vi "Radio Button Value.vi"(8 "Error In":errorcluster, 10 "Radio Buttons 2":refnum<vi>) -> (0 "Error Out":errorcluster, 2 "1st Value Selected?":bool)   [LabVIEW 2016]
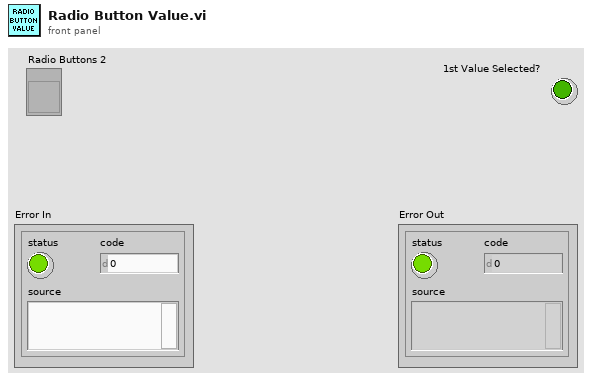
[diagram p1: front panel]
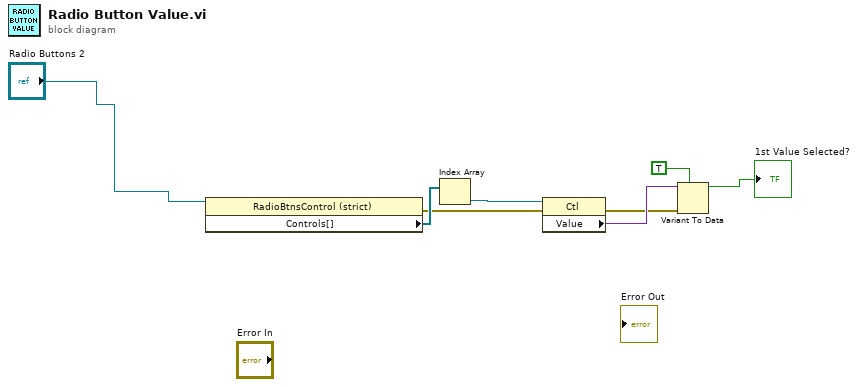
[diagram p0: block diagram]
diagram:
  n1 = property class="RadioBtnsControl (strict)"(reference="Radio Buttons 2") -> (error out=w4:errorcluster, "Controls[]"=w8:refnum<vi>[])  [unwired: 1 in, 1 out]
  n2 = Index Array(array=w8) -> (element=w7:refnum<vi>)  [unwired: 1 in]
  n3 = property class="Ctl"(reference=w7, error in=w4) -> (error out=w3:errorcluster, "Value"=w6:variant)  [unwired: 1 out]
  n4 = Variant To Data(error in=w3, type=TRUE, Variant=w6) -> (data=→"1st Value Selected?":bool)  [unwired: 1 out]
